vi "Global settings procedura tors.vi"() -> ()   [LabVIEW 2019]
panel:
  in  "settings procedura tors":T1={"rpm max"=0.0, "Impostazioni procedura"={"STEP RPM"=100.0, "TEMPO DI\nSTABILIZZAZIONE [s]"=10.0}}
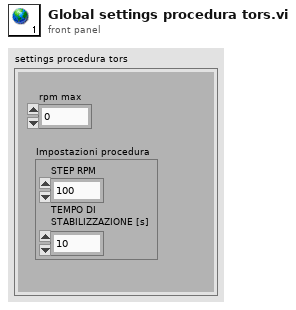
[diagram p1: front panel]
types:
  T1 = cluster{"rpm max":dbl, "Impostazioni procedura":cluster{"STEP RPM":dbl, "TEMPO DI\nSTABILIZZAZIONE [s]":dbl}}
diagram:
